vi "test Write and Read U32.vi"(8 "error in (no error)":errorcluster, 11 "TestCase in":refnum<class "Read Value Tests.lvclass">) -> (0 "error out":errorcluster, 3 "TestCase out":refnum<class "Read Value Tests.lvclass">)   [LabVIEW 2017, in "Read Value Tests.lvclass"]
uses:
  Read Value Tests.lvclass
  <vilib>/NI/Memory Manager/Classes/Pointer/Pointer.lvclass/Pointer.ctl
  <vilib>/NI/Memory Manager/Classes/Pointer/Protected/Parameter Checking/Check Null Pointer.vi
  <vilib>/NI/Memory Manager/Classes/Pointer/Private/Deallocate.vi
  <vilib>/NI/Memory Manager/Classes/Pointer/Protected/Errors.vi
  <vilib>/NI/Memory Manager/Classes/Pointer/Protected/Error VIs/Null Pointer.vi
  <vilib>/NI/Memory Manager/Classes/Pointer/API/Accessors/Get Address.vi
  <vilib>/NI/Memory Manager/Classes/Pointer/Protected/Get Internal.vi
  <vilib>/NI/Memory Manager/Classes/Pointer/Protected/Error VIs/Zone.vi
  <vilib>/NI/Memory Manager/Classes/Pointer/API/Accessors/Set Address.vi
  <vilib>/NI/Memory Manager/Classes/Pointer/API/Accessors/Set Size.vi
  <vilib>/NI/Memory Manager/Classes/Pointer/Private/Set Internal.vi
  <vilib>/NI/Memory Manager/Classes/Pointer/Protected/Error Building/Create Error.vi
  <vilib>/NI/Memory Manager/Constants/Constants.vi
  <vilib>/NI/Memory Manager/Constants/Library Name.vi
  <vilib>/NI/Memory Manager/Classes/Pointer/Protected/Error Building/Get Error Info.vi
  <vilib>/NI/Memory Manager/VIs/Write String into Source.vi
  <vilib>/NI/Memory Manager/VIs/Create Error Cluster.vi
  <vilib>/NI/Memory Manager/VIs/VIs for Poly/Create Error Cluster (256B).vi
  <vilib>/NI/Memory Manager/VIs/Set Error Status.vi
  <vilib>/NI/Memory Manager/VIs/Set Error Code.vi
  <vilib>/NI/Memory Manager/VIs/Set Error Source.vi
  Engine/Classes/Buffer/Buffer.lvclass
  C:/Program Files (x86)/National Instruments/LabVIEW 2017/vi.lib/NI/Memory Manager/Classes/Pointer/Pointer.lvclass
  Engine/Classes/Buffer/Read 0D U32.vi
  <vilib>/addons/_JKI Toolkits/VI Tester/TestCase.llb/TestCase.lvclass
  <vilib>/NI/Memory Manager/Classes/Pointer/Pointer.lvclass
  C:/Program Files (x86)/National Instruments/LabVIEW 2017/vi.lib/addons/_JKI Toolkits/VI Tester/TestCase.llb/TestCase.lvclass
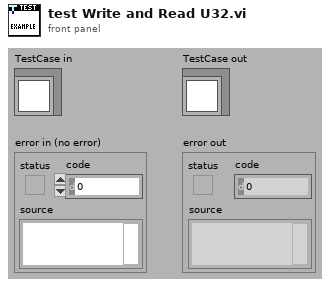
[diagram p1: front panel]
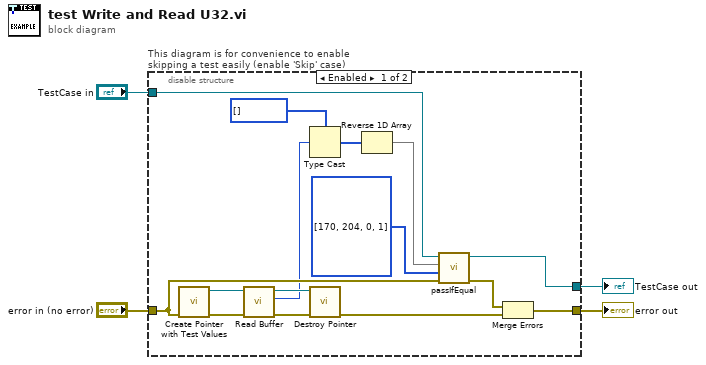
[diagram p0: block diagram]
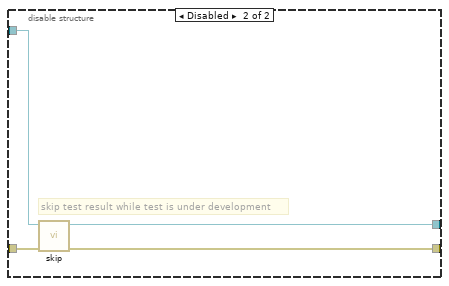
[diagram p2: hidden frame]
diagram:
  n1 = disable-structure "This diagram is for convenience to enable skipping a test easily (enable 'Skip' case)" shown="Enabled" {
    disable-tunnel: "TestCase in" -> [w11 w23]
    disable-tunnel: [w14 w21] -> w1
    disable-tunnel: [w9 w22] -> w2
    disable-tunnel: "error in (no error)" -> [w10 w20]
    frame Enabled {
      n2 = call "Create Pointer with Test Values.vi"("error in (no error)"=w10) -> ("error out"=w7:errorcluster, "Buffer out"=w5:refnum<class "Buffer.lvclass">)  [unwired: 9 in]
      n3 = call-poly "Read Buffer.vi"("error in (no error)"=w7, "Buffer in"=w5) -> ("error out"=w18:errorcluster, "value out"=w8:u32, "Buffer out"=w19:refnum<class "Buffer.lvclass">)  [unwired: 6 in, 1 out]
      n4 = Type Cast(type=u8[] [] ("buffer in"), x=w8) -> (*(type *) &x=w17:u8[])
      n5 = call <vilib>:"Destroy Pointer.vi"("error in (no error)"=w18, "Pointer in"=w19) -> ("error out"=w6:errorcluster)  [unwired: 8 in, 1 out]
      n6 = Reverse 1D Array(array=w17) -> (reversed array=w12:u8[])
      n7 = call-dynamic "passIfEqual.vi"("error in (no error)"=w10, "y"=u8[] [170, 204, 0, 1] ("subarray 2"), "x"=w12, "TestCase in"=w11) -> ("error out"=w15:errorcluster, "TestCase out"=w14:refnum<class "Read Value Tests.lvclass">)  [unwired: 6 in]
      n8 = Merge Errors(w15, w6) -> (w9:errorcluster)
    }
    frame Disabled {
      # "skip test result while test is under development"
      n9 = call <vilib>:"skip.vi"("error in (no error)"=w20, "TestCase in"=w23) -> ("error out"=w22:errorcluster, "TestCase out"=w21:refnum<class "Read Value Tests.lvclass">)  [unwired: 8 in]
    }
  }
  "error out" <- w2
  "TestCase out" <- w1
